vi "LocalWaypointEncode.vi"(1 "LocalWaypointRec":T1) -> (0 "Array":u8[](array[numeric]))   [LabVIEW 2009]
uses:
  LocalWaypointRec.ctl
panel:
  out "output":string
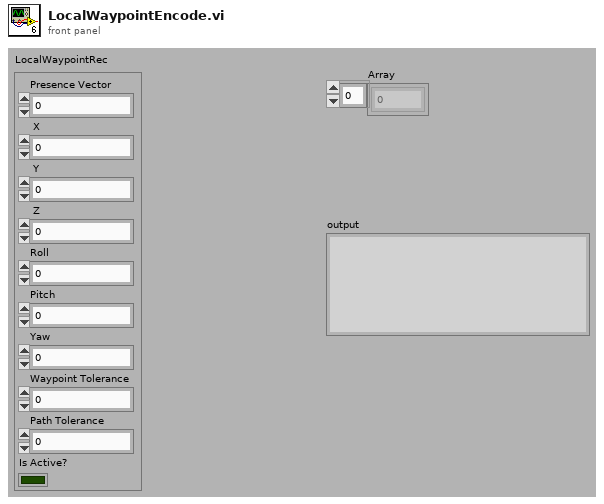
[diagram p1: front panel]
types:
  T1 = typedef "LocalWaypointRec.ctl" = cluster{"Presence Vector":u8, " X":dbl, " Y":dbl, " Z":dbl, "Roll":dbl, "Pitch":dbl, "Yaw":dbl, "Waypoint Tolerance":dbl, "Path Tolerance":dbl, "Is Active?":bool}
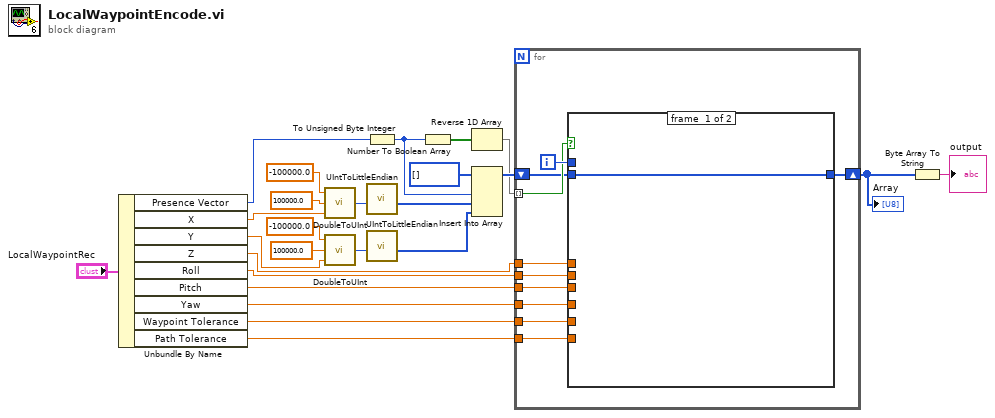
[diagram p0: block diagram]
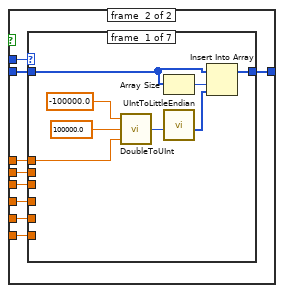
[diagram p2: hidden frame]
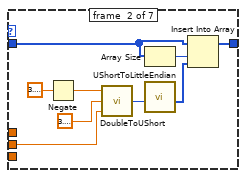
[diagram p3: hidden frame]
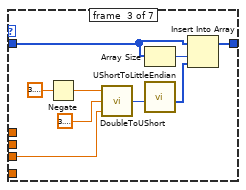
[diagram p4: hidden frame]
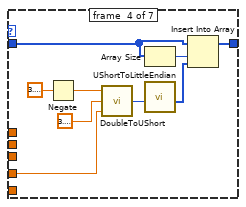
[diagram p5: hidden frame]
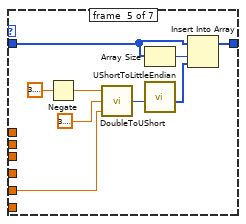
[diagram p6: hidden frame]
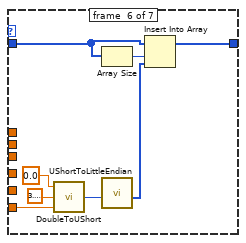
[diagram p7: hidden frame]
diagram:
  n1 = Unbundle By Name("LocalWaypointRec") -> ("Presence Vector"=w19:u8, "X"=w14:dbl, "Y"=w10:dbl, "Z"=w25:dbl, "Roll"=w24:dbl, "Pitch"=w23:dbl, "Yaw"=w22:dbl, "Waypoint Tolerance"=w21:dbl, "Path Tolerance"=w20:dbl)
  n2 = call "DoubleToUInt.vi"("Value"=w14, "Max"=100000.0, "Min"=-100000.0) -> ("scaled Integer"=w15:u32)
  n3 = call "DoubleToUInt.vi"("Value"=w10, "Max"=100000.0, "Min"=-100000.0) -> ("scaled Integer"=w11:u32)
  n4 = To Unsigned Byte Integer(number=w19) -> (unsigned 8bit integer=w3:u8)
  n5 = call "UIntToLittleEndian.vi"("Number"=w15) -> ("byte array"=w1:u8[])  [unwired: 10 in]
  n6 = call "UIntToLittleEndian.vi"("Number"=w11) -> ("byte array"=w2:u8[])  [unwired: 10 in]
  n7 = Number To Boolean Array(number=w3) -> (Boolean array=w5:bool[])
  n8 = Reverse 1D Array(array=w5) -> (reversed array=w4:bool[])
  n9 = Insert Into Array(array=u8[] [], new element #1=w3, new element #2=w1, new element #3=w2) -> (w8:u8[])  [unwired: 1 in]
  n10 = for {
    tunnel: w25 -> [w34]
    tunnel: w24 -> [w33]
    tunnel: w23 -> [w32]
    tunnel: w22 -> [w31]
    tunnel: w21 -> [w30]
    tunnel: w20 -> [w29]
    tunnel: w4 -> [w28] mode=indexing
    shift-right: [w27] -> w7
    shift-left: w8 -> [w26]
    i -> [w35]
    n11 = case shown="False" w28 {
      tunnel: w35 -> [_ w45]
      tunnel: w34 -> [_ w44]
      tunnel: w33 -> [_ w43]
      tunnel: w32 -> [_ w42]
      tunnel: w31 -> [_ w41]
      tunnel: w30 -> [_ w40]
      tunnel: w29 -> [_ w39]
      tunnel: [w36 w38] -> w27
      tunnel: w26 -> [w36 w37]
      frame #0 {
      }
      frame #1 {
        n12 = case shown="3" w45 {
          tunnel: w44 -> [w49 _ _ _ _ _ _]
          tunnel: w43 -> [_ w59 _ _ _ _ _]
          tunnel: w42 -> [_ _ w66 _ _ _ _]
          tunnel: w41 -> [_ _ _ w75 _ _ _]
          tunnel: w40 -> [_ _ _ _ w84 _ _]
          tunnel: w39 -> [_ _ _ _ _ w93 _]
          tunnel: [w48 w62 w65 w74 w83 w92 w98] -> w38
          tunnel: w37 -> [w47 w55 w64 w73 w82 w91 w98]
          frame #0 {
            n13 = call "DoubleToUInt.vi"("Value"=w49, "Max"=100000.0, "Min"=-100000.0) -> ("scaled Integer"=w51:u32)
            n14 = Array Size(array=w47) -> (size(s)=w46:i32)
            n15 = call "UIntToLittleEndian.vi"("Number"=w51) -> ("byte array"=w50:u8[])  [unwired: 10 in]
            n16 = Insert Into Array(array=w47, index=w46, new element=w50) -> (w48:u8[])
          }
          frame #1 {
            n17 = Negate(x=3.141592653589793) -> (-x=w58:dbl)
            n18 = call "DoubleToUShort.vi"("Value"=w59, "Max"=3.141592653589793, "Min"=w58) -> ("scaled Integer"=w56:u16)
            n19 = Array Size(array=w55) -> (size(s)=w54:i32)
            n20 = call "UShortToLittleEndian.vi"("Number"=w56) -> ("byte array"=w60:u8[])  [unwired: 10 in]
            n21 = Insert Into Array(array=w55, index=w54, new element=w60) -> (w62:u8[])
          }
          frame #2 {
            n22 = Negate(x=3.141592653589793) -> (-x=w67:dbl)
            n23 = call "DoubleToUShort.vi"("Value"=w66, "Max"=3.141592653589793, "Min"=w67) -> ("scaled Integer"=w71:u16)
            n24 = Array Size(array=w64) -> (size(s)=w63:i32)
            n25 = call "UShortToLittleEndian.vi"("Number"=w71) -> ("byte array"=w70:u8[])  [unwired: 10 in]
            n26 = Insert Into Array(array=w64, index=w63, new element=w70) -> (w65:u8[])
          }
          frame #3 {
            n27 = Negate(x=3.141592653589793) -> (-x=w77:dbl)
            n28 = call "DoubleToUShort.vi"("Value"=w75, "Max"=3.141592653589793, "Min"=w77) -> ("scaled Integer"=w80:u16)
            n29 = Array Size(array=w73) -> (size(s)=w72:i32)
            n30 = call "UShortToLittleEndian.vi"("Number"=w80) -> ("byte array"=w79:u8[])  [unwired: 10 in]
            n31 = Insert Into Array(array=w73, index=w72, new element=w79) -> (w74:u8[])
          }
          frame #4 {
            n32 = Negate(x=3.141592653589793) -> (-x=w86:dbl)
            n33 = call "DoubleToUShort.vi"("Value"=w84, "Max"=3.141592653589793, "Min"=w86) -> ("scaled Integer"=w89:u16)
            n34 = Array Size(array=w82) -> (size(s)=w81:i32)
            n35 = call "UShortToLittleEndian.vi"("Number"=w89) -> ("byte array"=w88:u8[])  [unwired: 10 in]
            n36 = Insert Into Array(array=w82, index=w81, new element=w88) -> (w83:u8[])
          }
          frame #5 {
            n37 = call "DoubleToUShort.vi"("Value"=w93, "Max"=3.141592653589793, "Min"=0.0) -> ("scaled Integer"=w97:u16)
            n38 = Array Size(array=w91) -> (size(s)=w90:i32)
            n39 = call "UShortToLittleEndian.vi"("Number"=w97) -> ("byte array"=w96:u8[])  [unwired: 10 in]
            n40 = Insert Into Array(array=w91, index=w90, new element=w96) -> (w92:u8[])
          }
          frame #6 {
          }
        }
      }
    }
  }
  "Array" <- w7
  n41 = Byte Array To String(unsigned byte array=w7) -> (string=→"output":string)
